vi "OverlayRectangleBoundingBox.vi"(6 "Color":u32(colorbox)=16711680, 7 "GroupName":string, 8 "error in":errorcluster, 9 "Drawing Mode (Frame)":T2, 10 "Rectangle":T1, 11 "Image Reference In":T3) -> (0 "error out":errorcluster, 3 "Image Reference Out":T3)   [LabVIEW 2020, in "OpenLvVision_Overlays.lvlib"]
doc: "Overlays an rectangle on top of an image.\nDraws it by the given bounding box coordinates."
uses:
  OpenLvVision_Overlays.lvlib
  <vilib>/OpenLvVision/OpenLvVision_Image/Management/TypeDef/OLV Image.ctl
  <vilib>/OpenLvVision/OpenLvVision_Image/Management/OLV Management.lvlib
  TypeDefs/DrawingMode.ctl
  <vilib>/OpenLvVision/OpenLvVision_Image/DataAccess/TypeDef/OLV RectangleI32.ctl
  <vilib>/OpenLvVision/OpenLvVision_Image/DataAccess/OLV DataAccess.lvlib
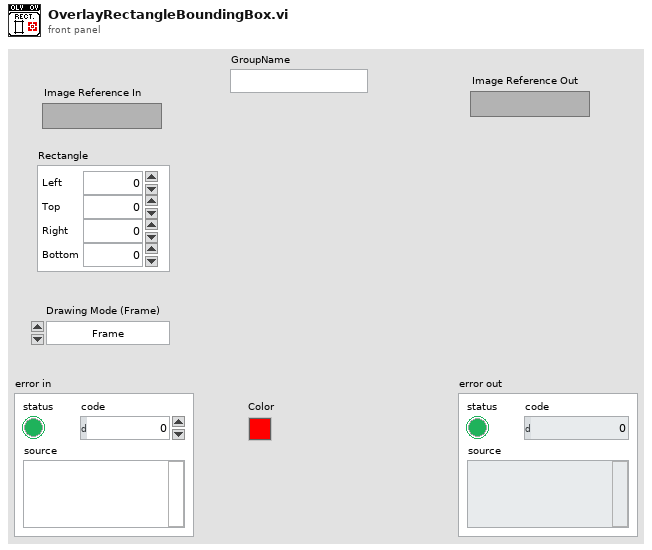
[diagram p1: front panel]
types:
  T1 = typedef "OLV OpenLvVision_Image.lvlib/OLV DataAccess.lvlib/OLV RectangleI32.ctl" = cluster{"Left":i32, "Top":i32, "Right":i32, "Bottom":i32}
  T2 = typedef "OpenLvVision_Overlays.lvlib/DrawingMode.ctl" = enum16{"Frame", "Fill"}
  T3 = typedef "OLV OpenLvVision_Image.lvlib/OLV Management.lvlib/OLV Image.ctl" = refnum<image>
  T4 = typedef "IMAQ Image.ctl" = refnum<image>
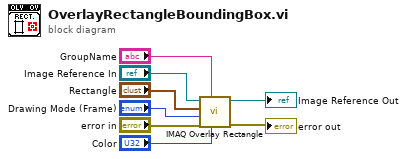
[diagram p0: block diagram]
diagram:
  n1 = call "IMAQ Overlay Rectangle"("Color"="Color", "Group"="GroupName", "error in (no error)"="error in", "Drawing Mode (Frame)"="Drawing Mode (Frame)", "Rectangle"="Rectangle", "Image"="Image Reference In") -> ("error out"=→"error out":errorcluster, "Image Out"=→"Image Reference Out":T4)  [unwired: 4 in]
